vi "SMO.Control Experiment.GetPrivateEvents.vi"(8 "error in (no error)":errorcluster, 11 "Control Experiment":refnum<class "SMO.Control Experiment.lvclass">) -> (0 "error out":errorcluster, 2 "Private Events":T1, 3 "Control Experiment out":refnum<class "SMO.Control Experiment.lvclass">)   [LabVIEW 2019, in "SMO.Control Experiment.lvclass"]
doc: "---------------------------------------------------------------\nJKI State Machine Objects™\nhttp://jki.net/state-machine-objects/\nCopyright (C) 2005-2015, JKI <info@jki.net>\nALL RIGHTS RESERVEDJKI State Machine Objects (SMO) 1.0.0.4\nJKI - JKI\nCopyright (c) 2015, JKI"
uses:
  SMO.Control Experiment.lvclass
  Typedefs/PrivateEvents--Cluster.ctl
  Typedefs/PrivateEvents--SMO.Control Experiment.saveKHpreset.ctl
  Typedefs/PrivateEvents--SMO.Control Experiment.setUIconfig.ctl
  SMO.Control Experiment UI/Typedefs/UI Config--Cluster.ctl
  SMO.Control Experiment UI/Typedefs/UI Channels--Cluster.ctl
  SMO.Control Experiment UI/Typedefs/UI Channels.AI--Cluster.ctl
  SMO.Control Experiment UI/Typedefs/UI Channels.Device--Cluster.ctl
  Control Experiment/Typedefs/KH Mode-enum.ctl
  SMO.Control Experiment UI/Typedefs/UI Channels.KH--Cluster.ctl
  <userlib>/LevyLab/Krohn Hite 7008/typedefs/Input Configuration-Enum.ctl
  <userlib>/LevyLab/Krohn Hite 7008/typedefs/Gain-Enum.ctl
  <userlib>/LevyLab/Krohn Hite 7008/typedefs/Shunt-Enum.ctl
  SMO.Control Experiment UI/Typedefs/UI Channels.AO--Cluster.ctl
  Control Experiment/Typedefs/Instrument--enum.ctl
  <userlib>/LevyLab/Krohn Hite 7008/typedefs/Coupling-Enum.ctl
  <userlib>/LevyLab/Krohn Hite 7008/typedefs/Filter-Enum.ctl
  Typedefs/PrivateEvents--SMO.Control Experiment.loadKHpreset.ctl
  SMO.Control Experiment.lvclass/SMO.Control Experiment.ctl
  SMO.Control Experiment UI/SMO.Control Experiment UI.lvclass
  Control Experiment/Control Experiment.lvclass
  <userlib>/LevyLab/Krohn Hite 7008/Instrument.KH7008.lvclass
panel:
  # "For instructions on how to use the JKI State Machine Objects, examples and video tutorials, visit:\nhttp://jki.net/state-machine-objects/\n\nJKI State Machine Objects™\nhttp://jki.net/state-machine-objects/\nCopyright (C) 2005-2015, JKI <info@jki.net>\nALL RIGHTS RESERVED"
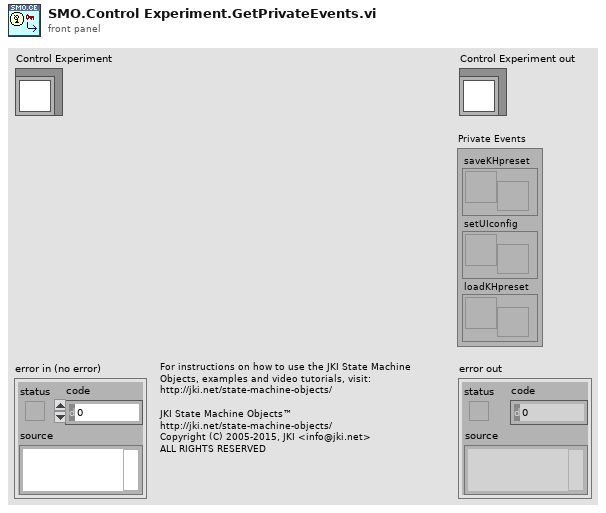
[diagram p1: front panel]
types:
  T1 = typedef "SMO.Control Experiment.lvclass/PrivateEvents--Cluster.ctl" = cluster{"saveKHpreset":refnum<user-event>, "setUIconfig":refnum<user-event>, "loadKHpreset":refnum<user-event>}
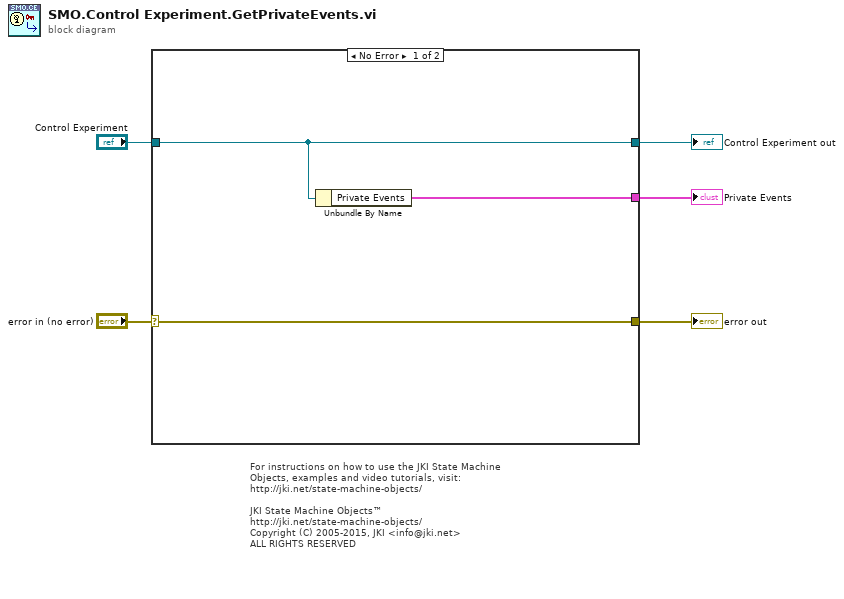
[diagram p0: block diagram]
diagram:
  # "For instructions on how to use the JKI State Machine Objects, examples and video tutorials, visit:\nhttp://jki.net/state-machine-objects/\n\nJKI State Machine Objects™\nhttp://jki.net/state-machine-objects/\nCopyright (C) 2005-2015, JKI <info@jki.net>\nALL RIGHTS RESERVED"
  n1 = case shown="No Error" "error in (no error)" {
    selector: "error in (no error)" -> [w7 w9]
    tunnel: "Control Experiment" -> [w6 w10]
    tunnel: [w7 w9] -> w4
    tunnel: [w6 w10] -> w3
    tunnel: [w8 _] -> w1
    frame No Error {
      n2 = Unbundle By Name(w6) -> ("Private Events"=w8:T1)
    }
    frame Error {
    }
  }
  "error out" <- w4
  "Control Experiment out" <- w3
  "Private Events" <- w1
